vi "Set Custom Bitfile.vi"(8 "error in (no error)":errorcluster, 11 "Custom FPGA Reference In":T1) -> (0 "error out":errorcluster, 3 "Custom FPGA Reference Out":T1)   [LabVIEW 2021, in "Utilities.lvlib"]
doc: "Sets a custom FPGA reference."
uses:
  <vilib>/myRIO/Instrument Drivers/Utilities/Utilities.lvlib
  <vilib>/myRIO/Common/Instrument Driver Framework/Utilities/typedefs/Generic FPGA Reference.ctl
  <vilib>/myRIO/Common/Instrument Driver Framework/Utilities/typedefs/FPGA Ref Manager Action Enum.ctl
  <vilib>/myRIO/Common/Instrument Driver Framework/Utilities/typedefs/Ref Counter Action Enum.ctl
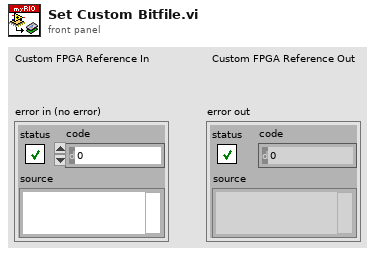
[diagram p1: front panel]
types:
  T1 = typedef "Generic FPGA Reference.ctl" = refnum<k20>
  T2 = typedef "FPGA Ref Manager Action Enum.ctl" = enum16{"Get", "Set", "Reset"}
  T3 = typedef "Ref Counter Action Enum.ctl" = enum16{"Set", "Get", "Increment", "Decrement"}
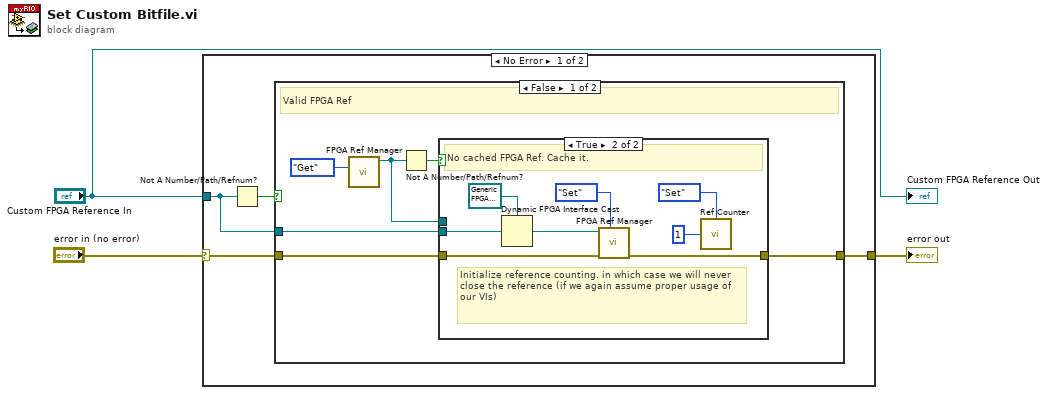
[diagram p0: block diagram]
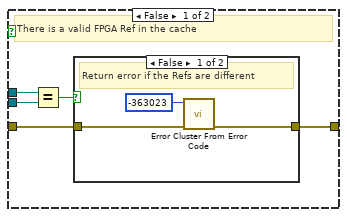
[diagram p2: hidden frame]
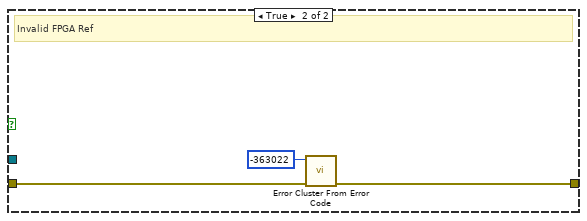
[diagram p4: hidden frame]
diagram:
  n1 = case shown="No Error" "error in (no error)" {
    selector: "error in (no error)" -> [w4 w34]
    tunnel: "Custom FPGA Reference In" -> [w6 _]
    tunnel: [w5 w34] -> w2
    frame No Error {
      n2 = Not A Number/Path/Refnum?(number/path/refnum=w6) -> (NaN/Path/Refnum?=w7:bool)
      n3 = case shown="False" w7 {
        tunnel: w4 -> [w11 w32]
        tunnel: [w13 w33] -> w5
        tunnel: w6 -> [w10 _]
        frame False {
          # "Valid FPGA Ref"
          n4 = call <vilib>:"FPGA Ref Manager.vi"("Action"=FPGA_Ref_Manager_Action_Enum."Get") -> ("Generic FPGA Reference out"=w8:T1)  [unwired: 8 in, 1 out]
          n5 = Not A Number/Path/Refnum?(number/path/refnum=w8) -> (NaN/Path/Refnum?=w9:bool)
          n6 = case shown="True" w9 {
            tunnel: [w17 w30] -> w13
            tunnel: w11 -> [w18 w27]
            tunnel: w10 -> [w16 w26]
            tunnel: w8 -> [w15 _]
            frame False {
              # "There is a valid FPGA Ref in the cache"
              n7 = Equal?(x=w15, y=w16) -> (x = y?=w14:bool)
              n8 = case shown="False" w14 {
                tunnel: w18 -> [w20 w22]
                tunnel: [w19 w22] -> w17
                frame False {
                  # "Return error if the Refs are different"
                  n9 = call <vilib>:"Error Cluster From Error Code.vi"("error in (no error)"=w20, "error code (0)"=-363023) -> ("error out"=w19:errorcluster)  [unwired: 7 in]
                }
                frame True {
                  # "Do nothing if the Refs are same"
                }
              }
            }
            frame True {
              # "Initialize reference counting. in which case we will never close the reference (if we again assume proper usage of our VIs)"
              # "No cached FPGA Ref. Cache it."
              n10 = Dynamic FPGA Interface Cast(Session In=T1 refnum ("Generic FPGA Reference"), Type=w26) -> (Session Out=w25:T1)
              n11 = call <vilib>:"FPGA Ref Manager.vi"("Action"=FPGA_Ref_Manager_Action_Enum."Set", "error in (no error)"=w27, "Generic FPGA Reference in"=w25) -> ("error out"=w30:errorcluster)  [unwired: 6 in, 1 out]
              n12 = call <vilib>:"Ref Counter.vi"("Ref Count in"=u32 1 ("RefCount in"), "Ref Counter Action Enum"=Ref_Counter_Action_Enum."Set") -> ()  [unwired: 1 out]
            }
          }
        }
        frame True {
          # "Invalid FPGA Ref"
          n13 = call <vilib>:"Error Cluster From Error Code.vi"("error in (no error)"=w32, "error code (0)"=-363022) -> ("error out"=w33:errorcluster)  [unwired: 7 in]
        }
      }
    }
    frame Error {
    }
  }
  "error out" <- w2
  "Custom FPGA Reference Out" <- "Custom FPGA Reference In"
